vi "Translator.Translate.Status.vi"   [LabVIEW 2015]
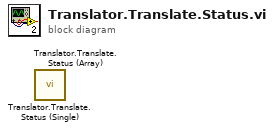
[diagram p0: block diagram]
diagram:
  n1 = call "Translator.Translate.Status (Single).vi"() -> ()  [unwired: 11 in, 1 out]
  n2 = call "Translator.Translate.Status (Array).vi"() -> ()  [unwired: 11 in, 1 out]
